vi "ExcelToATR Table (SubVI).vi"(10 "Shared_strings":string[][](array[string]), 11 "Table in":refnum<vi>) -> (0 "error out":errorcluster, 3 "TestArray":string[](array[string]))   [LabVIEW 2017]
uses:
  <vilib>/Utility/miscctls.llb/LVRowAndColumnTypeDef.ctl
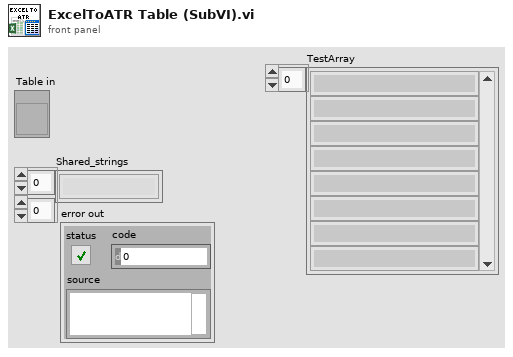
[diagram p1: front panel]
types:
  T1 = typedef "LVRowAndColumnTypeDef.ctl" = cluster{"Row":i32, "Column":i32}
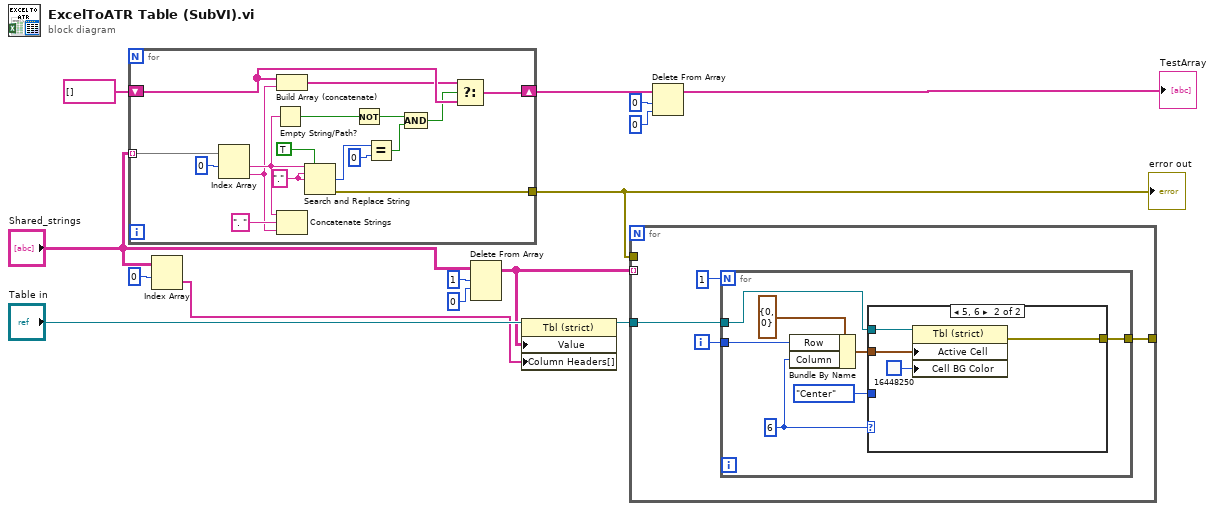
[diagram p0: block diagram]
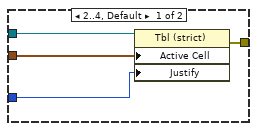
[diagram p2: hidden frame]
diagram:
  n1 = for {
    tunnel: "Shared_strings" -> [w17] mode=indexing
    shift-right: [w31] -> w4
    shift-left: string[] [] -> [w30]
    tunnel: [w29] -> w7
    w26 = "." ("search string")
    n2 = Index Array(array=w17, index #1=0 ("index")) -> (element #1=w16:string, element #2=w15:string)  [unwired: 1 in]
    n3 = Empty String/Path?(string/path=w16) -> (empty?=w25:bool)
    n4 = Build Array (concatenate)(w30, w15) -> (w19:string[])
    n5 = Concatenate Strings(w16, ". " ("string"), w15) -> ()  [unwired: 1 out]
    n6 = Search and Replace String(replace all?=TRUE ("replace all? (F)"), input string=w16, search string=w26, replace string=w26) -> (number of replacements=w24:i32, error out=w29:errorcluster)  [unwired: 4 in, 2 out]
    n7 = Not(x=w25) -> (.not. x?=w22:bool)
    n8 = Equal?(x=w24, y=0) -> (x = y?=w21:bool)
    n9 = Compound Arithmetic op=AND(w22, w21) -> (w20:bool)
    n10 = Select(t=w19, s=w20, f=w30) -> (s? t:f=w31:string[])
  }
  "error out" <- w7
  n11 = Index Array(array="Shared_strings", index (row)=0 ("length")) -> (element=w1:string[])  [unwired: 1 in]
  n12 = Delete From Array(array="Shared_strings", length=1, index (row)=0) -> (array with subset deleted=w2:string[][])  [unwired: 1 in, 1 out]
  n13 = property on="Property Node" class="Tbl (strict)"(reference="Table in", "Value"=w2, "Column Headers[]"=w1) -> (reference out=w8:refnum<vi>)  [unwired: 1 in, 1 out]
  n14 = for {
    tunnel: [w35] -> _
    tunnel: w8 -> [w33]
    tunnel: w2 -> [_] mode=indexing
    tunnel: w7 -> [_]
    i -> [w34]
    n15 = for {
      N: 1 -> [_]
      tunnel: [w40] -> w35
      tunnel: w34 -> [w39]
      tunnel: w33 -> [w38]
      w36 = 6
      n16 = Bundle By Name(cluster=T1 {"Row"=0, "Column"=0} ("Active Cell:Active Cell"), "Row"=w39, "Column"=w36) -> (w41:T1)
      n17 = case shown="5, 6" w36 {
        tunnel: w41 -> [w46 w50]
        tunnel: [w43 w48] -> w40
        tunnel: w38 -> [w45 w47]
        tunnel: enum16{"Left", "Center", "Right"}."Center" ("Active Cell:Cell Justification") -> [w44 _]
        frame 2..4, Default {
          n18 = property on="Property Node" class="Tbl (strict)"(reference=w45, "Active Cell"=w46, "Justify"=w44) -> (error out=w43:errorcluster)  [unwired: 1 in, 1 out]
        }
        frame 5, 6 {
          n19 = property on="Property Node" class="Tbl (strict)"(reference=w47, "Active Cell"=w50, "Cell BG Color"=u32 16448250) -> (error out=w48:errorcluster)  [unwired: 1 in, 1 out]
        }
      }
    }
  }
  n20 = Delete From Array(array=w4, length=0, index=0) -> (array with subset deleted=→"TestArray":string[])  [unwired: 1 out]
